vi "lvCopy.vi"(8 "error in (no error)":errorcluster, 11 "CommandLine":string[](array[string])) -> (0 "error out":errorcluster, 2 "test details":string)   [LabVIEW 2019]
uses:
  <userlib>/_OpenG.lib/file/file.llb/File Exists - Scalar__ogtk.vi
  <userlib>/_OpenG.lib/file/file.llb/Build Path - File Names Array__ogtk.vi
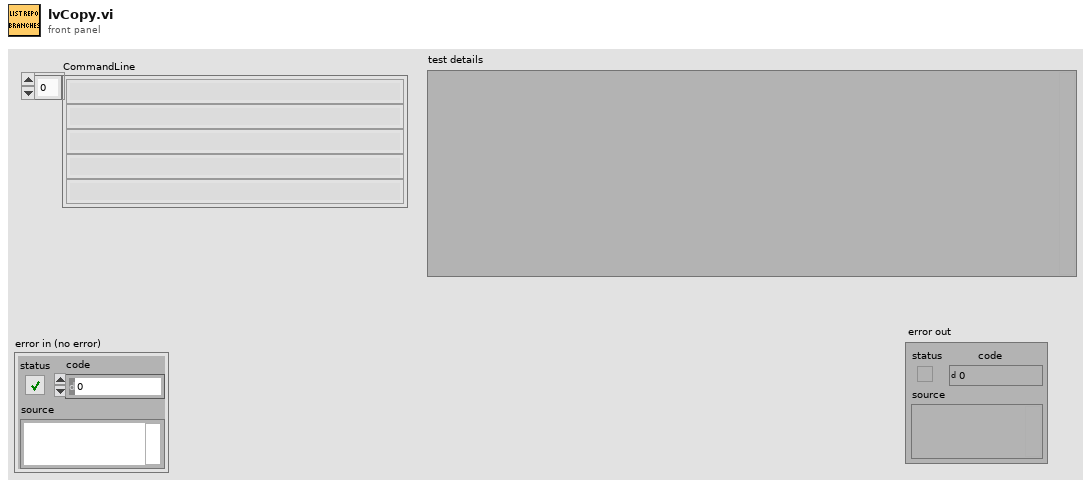
[diagram p1: front panel]
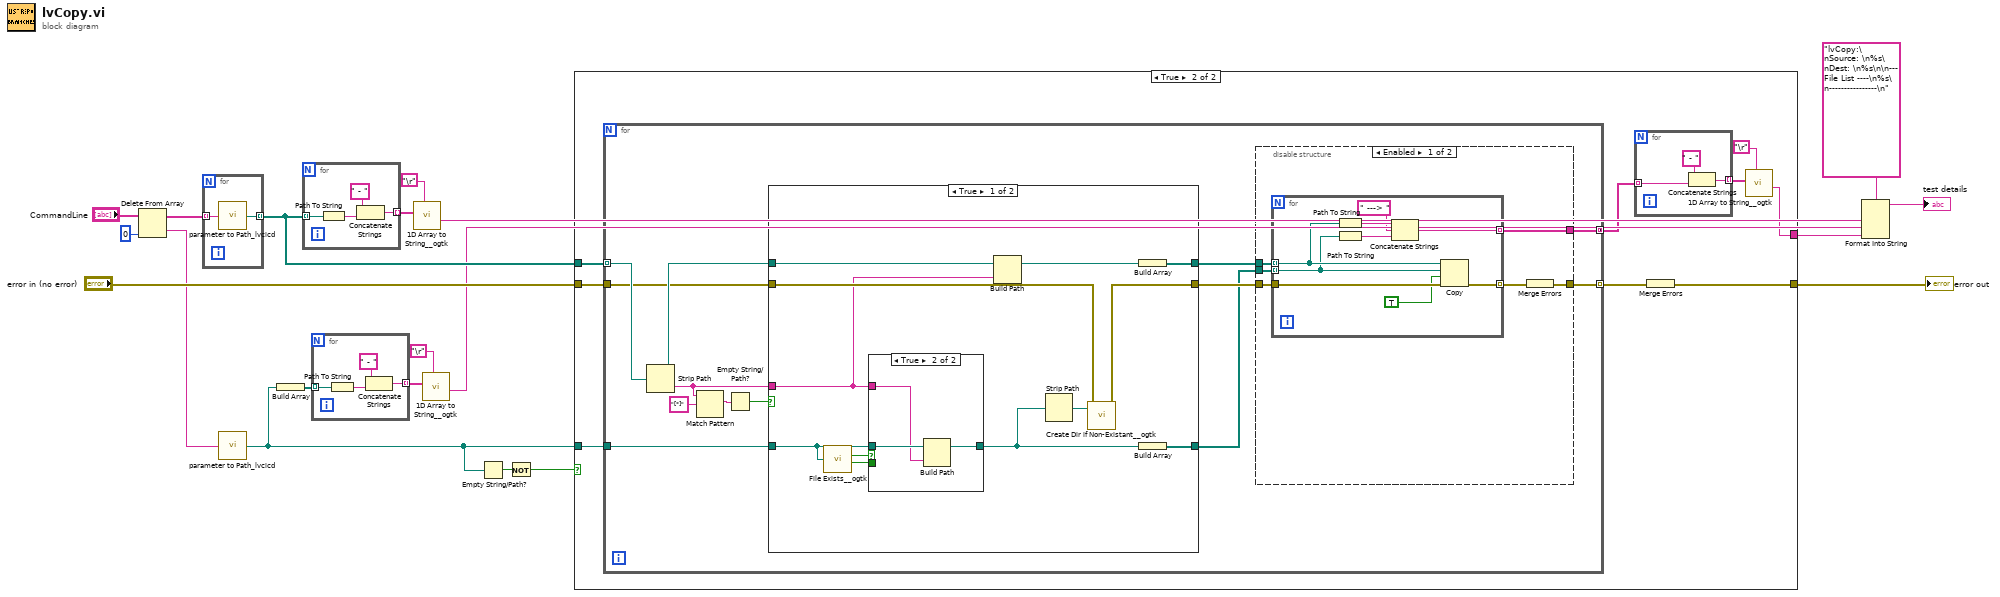
[diagram p0: block diagram]
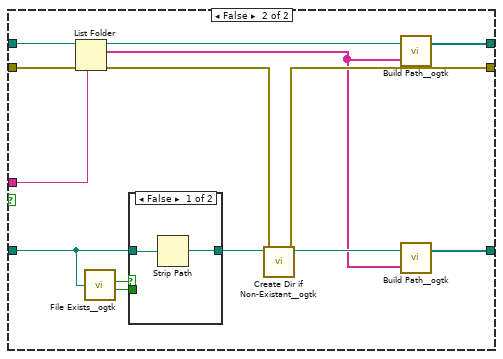
[diagram p4: hidden frame]
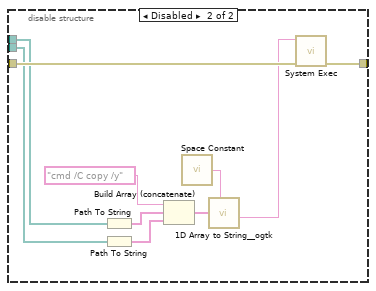
[diagram p6: hidden frame]
diagram:
  n1 = Delete From Array(array="CommandLine", index=0) -> (deleted portion=w12:string, array with subset deleted=w11:string[])  [unwired: 1 in]
  n2 = for {
    tunnel: [w22] -> w10 mode=indexing
    tunnel: w11 -> [w21] mode=indexing
    n3 = call "parameter to Path_lvcicd.vi"("String"=w21) -> ("Path"=w22:path)
  }
  n4 = call "parameter to Path_lvcicd.vi"("String"=w12) -> ("Path"=w2:path)
  n5 = Build Array(w2) -> (w3:path[])
  n6 = for {
    tunnel: w10 -> [w26] mode=indexing
    tunnel: [w23] -> w9 mode=indexing
    n7 = Path To String(path=w26) -> (string=w25:string)
    n8 = Concatenate Strings(" - " ("string"), w25) -> (w23:string)
  }
  n9 = for {
    tunnel: w3 -> [w30] mode=indexing
    tunnel: [w27] -> w4 mode=indexing
    n10 = Path To String(path=w30) -> (string=w29:string)
    n11 = Concatenate Strings(" - " ("string"), w29) -> (w27:string)
  }
  n12 = call <userlib>:"1D Array to String__ogtk.vi"("delimiter (Tab)"="\r", "Array of Strings"=w9) -> ("delimited string"=w7:string)  [unwired: 9 in]
  n13 = call <userlib>:"1D Array to String__ogtk.vi"("delimiter (Tab)"="\r", "Array of Strings"=w4) -> ("delimited string"=w1:string)  [unwired: 9 in]
  n14 = Empty String/Path?(string/path=w2) -> (empty?=w19:bool)
  n15 = Not(x=w19) -> (.not. x?=w17:bool)
  n16 = case shown="True" w17 {
    tunnel: "error in (no error)" -> [w31 w40]
    tunnel: [w31 w36] -> w20
    tunnel: w10 -> [_ w38]
    tunnel: w2 -> [_ w37]
    tunnel: [_ w33] -> w6
    frame False {
    }
    frame True {
      n17 = for {
        tunnel: w38 -> [w55] mode=indexing
        tunnel: w37 -> [w54]
        tunnel: w40 -> [w47]
        tunnel: [w56] -> w39 mode=indexing
        tunnel: [w44] -> w32 mode=concatenating
        n18 = Strip Path(path=w55) -> (stripped path=w49:path, name=w53:string)
        n19 = Match Pattern(string=w53, regular expression="[*]") -> (match substring=w51:string)  [unwired: 1 in, 3 out]
        n20 = Empty String/Path?(string/path=w51) -> (empty?=w50:bool)
        n21 = case shown="True" w50 {
          tunnel: w54 -> [w66 w80]
          tunnel: [w65 w83] -> w46
          tunnel: w53 -> [w59 w86]
          tunnel: w49 -> [w60 w85]
          tunnel: w47 -> [w62 w84]
          tunnel: [w61 w76] -> w48
          tunnel: [w57 w75] -> w45
          frame True {
            n22 = call-poly <userlib>:"File Exists__ogtk.vi"("file path"=w66) -> ("is directory"=w68:bool, "exists"=w67:bool)  [unwired: 6 in]
            n23 = case shown="True" w68 {
              tunnel: w67 -> [_ _]
              tunnel: w66 -> [w69 w72]
              tunnel: [w69 w71] -> w63
              tunnel: w59 -> [_ w70]
              frame False {
              }
              frame True {
                n24 = Build Path(base path=w72, name or relative path=w70) -> (appended path=w71:path)
              }
            }
            n25 = Build Path(base path=w60, name or relative path=w59) -> (appended path=w58:path)
            n26 = Strip Path(path=w63) -> (stripped path=w64:path)  [unwired: 1 out]
            n27 = call <userlib>:"Create Dir if Non-Existant__ogtk.vi"("error in (no error)"=w62, "Directory Path"=w64) -> ("error out"=w61:errorcluster)  [unwired: 7 in, 2 out]
            n28 = Build Array(w58) -> (w57:path[])
            n29 = Build Array(w63) -> (w65:path[])
          }
          frame False {
            n30 = List Folder(path=w85, pattern=w86, error in=w84) -> (path out=w74:path, filenames=w73:string[], error out=w77:errorcluster)  [unwired: 1 in, 1 out]
            n31 = call-poly <userlib>:"File Exists__ogtk.vi"("file path"=w80) -> ("is directory"=w82:bool, "exists"=w81:bool)  [unwired: 6 in]
            n32 = case shown="False" w82 {
              tunnel: w81 -> [_ _]
              tunnel: w80 -> [w88 w89]
              tunnel: [w87 w89] -> w79
              frame False {
                n33 = Strip Path(path=w88) -> (stripped path=w87:path)  [unwired: 1 out]
              }
              frame True {
              }
            }
            n34 = call <userlib>:"Create Dir if Non-Existant__ogtk.vi"("error in (no error)"=w77, "Directory Path"=w79) -> ("error out"=w76:errorcluster, "dup Directory Path"=w78:path)  [unwired: 7 in, 1 out]
            n35 = call-poly <userlib>:"Build Path__ogtk.vi"("name or relative path"=w73, "base path"=w74) -> ("appended path"=w75:path[])
            n36 = call-poly <userlib>:"Build Path__ogtk.vi"("name or relative path"=w73, "base path"=w78) -> ("appended path"=w83:path[])
          }
        }
        n37 = disable-structure shown="Enabled" {
          disable-tunnel: w48 -> [w95 w113]
          disable-tunnel: [w91 w114] -> w56
          disable-tunnel: w46 -> [w93 w111]
          disable-tunnel: w45 -> [w92 w112]
          disable-tunnel: [w90 _] -> w44
          frame Enabled {
            n38 = for {
              tunnel: w93 -> [w96] mode=indexing
              tunnel: w92 -> [w97] mode=indexing
              tunnel: w95 -> [w104]
              tunnel: [w103] -> w94 mode=indexing
              tunnel: [w101] -> w90 mode=indexing
              n39 = Path To String(path=w97) -> (string=w100:string)
              n40 = Path To String(path=w96) -> (string=w99:string)
              n41 = Concatenate Strings(w100, " ---> " ("string"), w99) -> (w101:string)
              n42 = Copy(8:w104, 9:TRUE ("overwrite (F)"), 10:w96, 11:w97) -> (0:w103:errorcluster)  [unwired: 1 in, 2 out]
            }
            n43 = Merge Errors(w94) -> (w91:errorcluster)
          }
          frame Disabled {
            n44 = Path To String(path=w112) -> (string=w109:string[])
            n45 = Path To String(path=w111) -> (string=w108:string[])
            n46 = Build Array (concatenate)("cmd /C copy /y" ("name"), w109, w108) -> (w107:string[])
            n47 = call <vilib>:"Space Constant.vi"() -> ("String"=w106:string)
            n48 = call <userlib>:"1D Array to String__ogtk.vi"("delimiter (Tab)"=w106, "Array of Strings"=w107) -> ("delimited string"=w105:string)  [unwired: 9 in]
            n49 = call <vilib>:"System Exec.vi"("error in (no error)"=w113, "command line"=w105) -> ("error out"=w114:errorcluster)  [unwired: 6 in, 3 out]
          }
        }
      }
      n50 = for {
        tunnel: [w42] -> w35 mode=indexing
        tunnel: w32 -> [w41] mode=indexing
        n51 = Concatenate Strings(" - " ("string"), w41) -> (w42:string)
      }
      n52 = Merge Errors(w39) -> (w36:errorcluster)
      n53 = call <userlib>:"1D Array to String__ogtk.vi"("delimiter (Tab)"="\r", "Array of Strings"=w35) -> ("delimited string"=w33:string)  [unwired: 9 in]
    }
  }
  "error out" <- w20
  n54 = Format Into String(format string="lvCopy:\nSource: \n%s\nDest: \n%s\n\n--- File List ----\n%s\n----------------\n", w7, w1, w6) -> (resulting string=→"test details":string)  [unwired: 2 in, 1 out]
